vi "Visa_Write read_UI SETPIN.vi"(0 "Serial Device in":refnum<class "Serial Device.lvclass">, 1 "VISA Refnum in":refnum<visa-resource-name>, 3 "Command to Send":string, 5 "error in (no error)":errorcluster) -> (14 "Serial Device out":refnum<class "Serial Device.lvclass">, 15 "VISA Refnum out":refnum<visa-resource-name>, 16 "Puerto":string, 17 "Valor Pin":string, 18 "Pin":bool, 19 "error out":errorcluster)   [LabVIEW 2020, in "Serial Device.lvclass"]
uses:
  Serial Device.lvclass
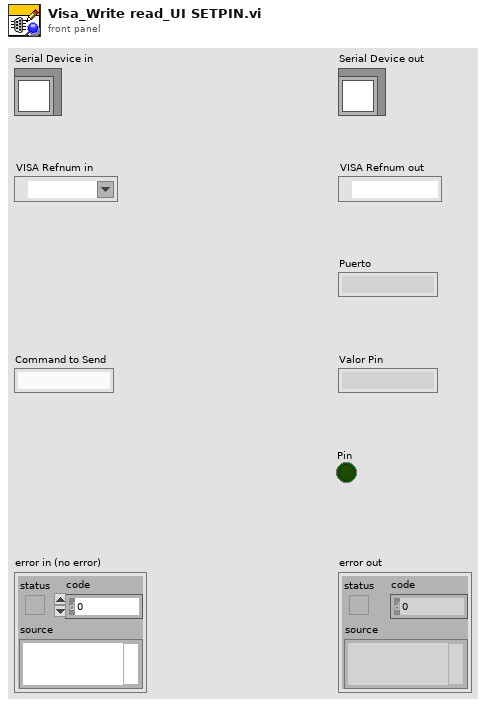
[diagram p1: front panel]
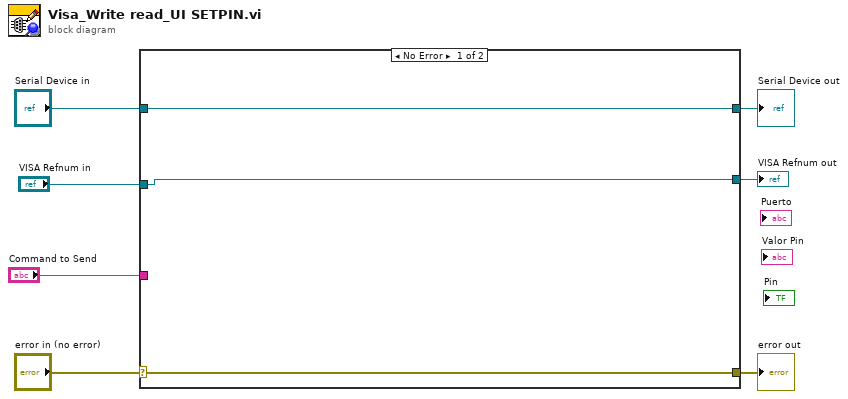
[diagram p0: block diagram]
diagram:
  n1 = case shown="No Error" "error in (no error)" {
    selector: "error in (no error)" -> [w9 w12]
    tunnel: [w9 w12] -> w6
    tunnel: [w10 w11] -> w4
    tunnel: "Serial Device in" -> [w10 w11]
    tunnel: "VISA Refnum in" -> [w8 _]
    tunnel: [w8 _] -> w2
    tunnel: "Command to Send" -> [_ _]
    frame No Error {
    }
    frame Error {
    }
  }
  "error out" <- w6
  "Serial Device out" <- w4
  "VISA Refnum out" <- w2
